vi "Read from Stream.vi"(10 "Stream in":refnum<class "Stream.lvclass">, 11 "Stream Formatter in":refnum<class "Stream Formatter.lvclass">) -> (0 "error out":errorcluster, 2 "Message Data":T1)   [LabVIEW 2020, in "Stream-Simple-Msg.lvlib" / "Stream Formatter.lvclass"]
uses:
  Stream Formatter.lvclass
  <vilib>/IlluminatedG/lv-stream/stream/Stream.lvclass
  Message/Message Data.ctl
  Message/Message___.lvclass
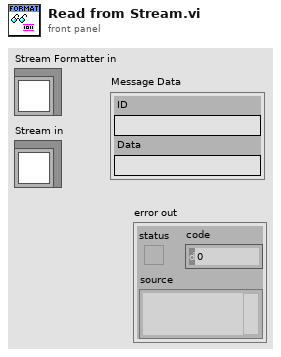
[diagram p1: front panel]
types:
  T1 = typedef "Stream-Simple-Msg.lvlib/Message___.lvclass/Message Data.ctl" = cluster{"ID":string, "Data":string}
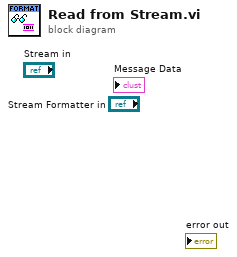
[diagram p0: block diagram]
diagram:
